vi "Write Settings.vi"(8 "error in":errorcluster, 10 "App Settings":T4, 11 "Controller in":refnum<class "Controller.lvclass">) -> (0 "error out":errorcluster, 3 "Controller out":refnum<class "Controller.lvclass">)   [LabVIEW 2022 SP3, in "Controller.lvlib" / "Controller.lvclass"]
uses:
  Controller.lvclass
  Typedefs/Storage Settings.ctl
  Typedefs/Image Formats.ctl
  Typedefs/PLC Settings.ctl
  Controller.lvclass/Controller.ctl
  <vilib>/Utility/config.llb/Write Key (U32).vi
  <vilib>/Utility/config.llb/Write Key (String).vi
  <vilib>/Utility/config.llb/Write Key (Path).vi
  <vilib>/Utility/config.llb/Write Key (Boolean).vi
  <vilib>/Utility/config.llb/NI_LVConfig.lvlib
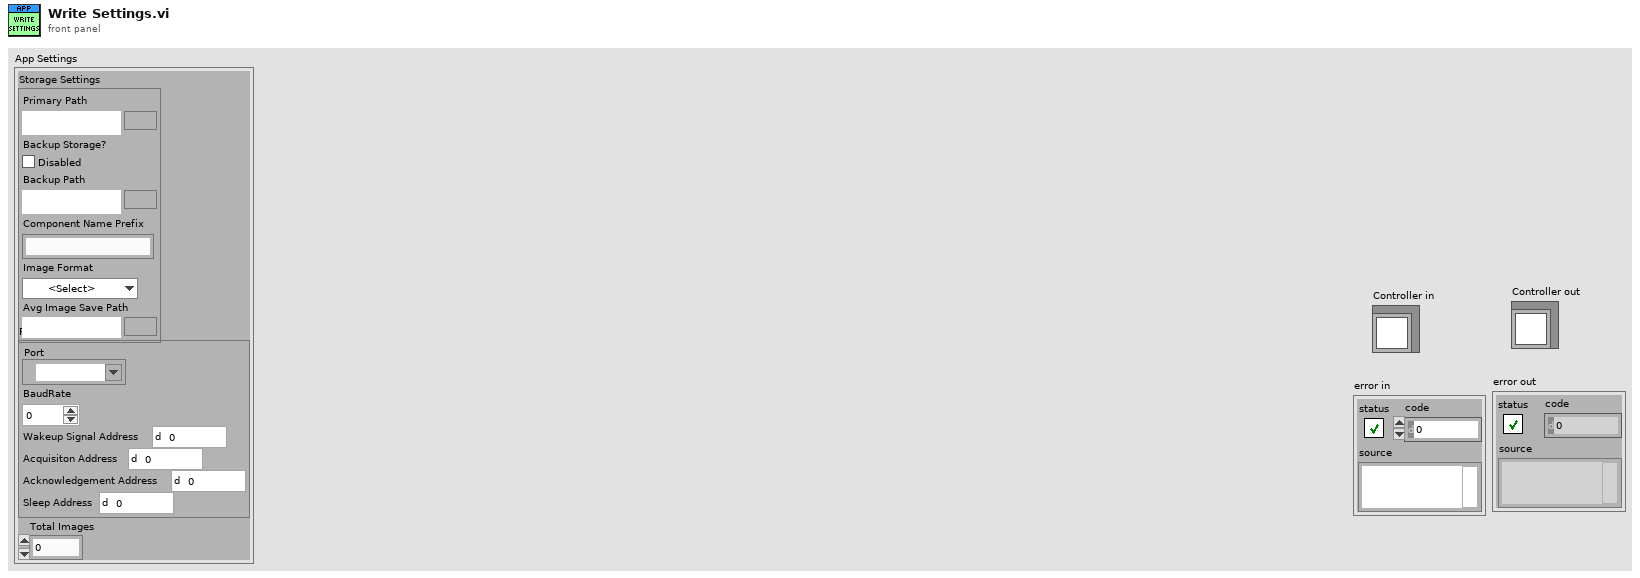
[diagram p1: front panel]
types:
  T1 = typedef "Storage Settings.ctl" = cluster{"Primary Path":path, "Backup Storage?":bool, "Backup Path":path, "Component Name Prefix":string, "Image Format":T2, "Avg Image Save Path":path}
  T2 = typedef "Image Formats.ctl" = enum16{"<Select>", "TIFF", "RAW"}
  T3 = typedef "PLC Settings.ctl" = cluster{"Port":refnum<visa-resource-name>, "BaudRate":u32, "Wakeup Signal Address ":u16, "Acquisiton Address":u16, "Acknowledgement Address":u16, "Sleep Address":u32}
  T4 = cluster{"Storage Settings":T1, "PLC Settings":T3, "Total Images":u32}
  T5 = cluster{"Config File ":path, "Configuration":path, "Event Log":path, "Error Log":path}
  T6 = typedef "NI_LVConfig.lvlib/Config Data RefNum.ctl" = refnum<k1>
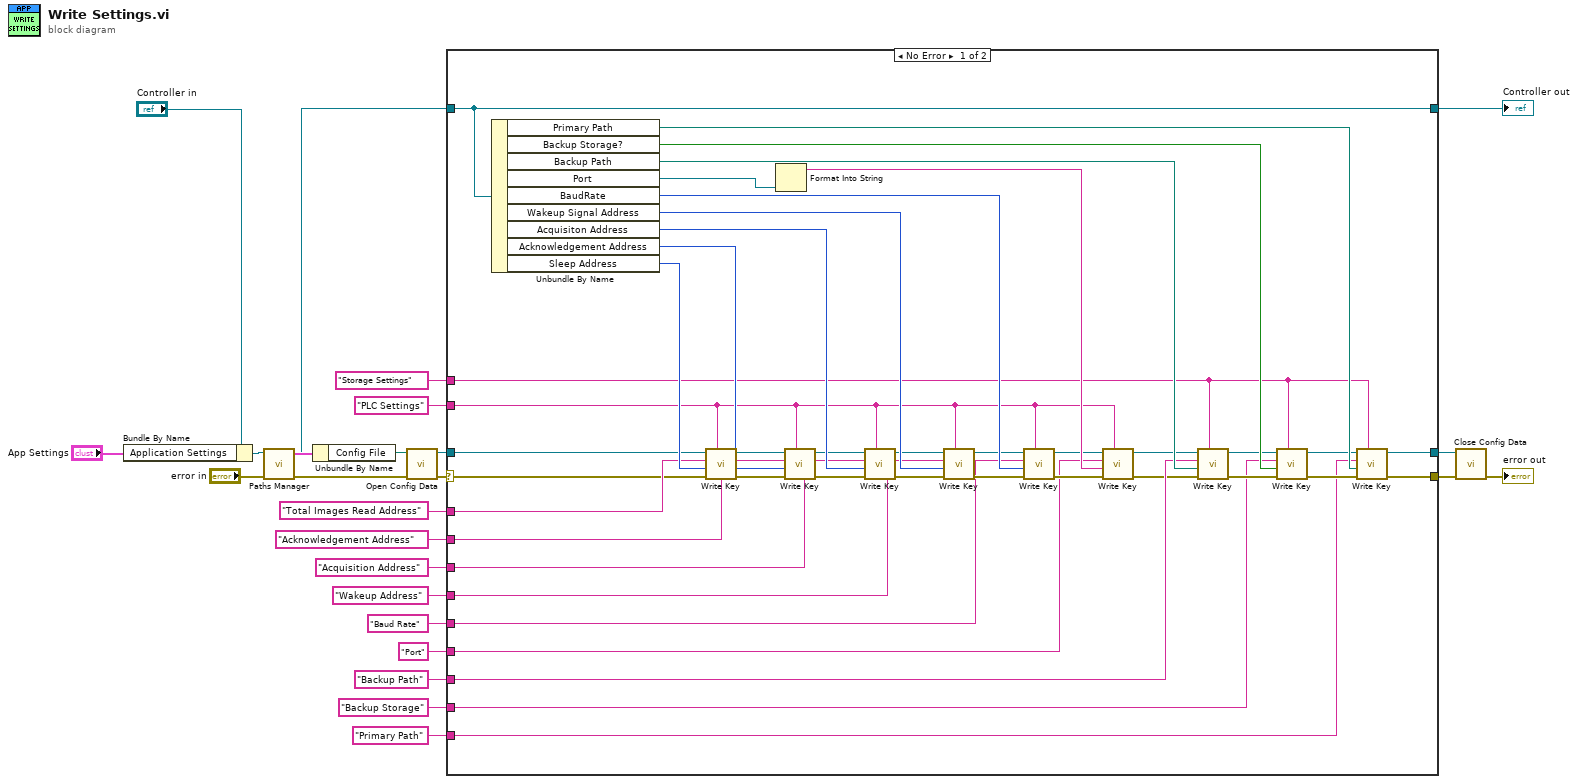
[diagram p0: block diagram]
diagram:
  n1 = Bundle By Name(cluster="Controller in", "Application Settings"="App Settings") -> (w2:refnum<class "Controller.lvclass">)
  n2 = call "Paths Manager.vi"("error in"="error in", "Controller in"=w2) -> ("error out"=w23:errorcluster, "Paths"=w21:T5, "Controller out"=w18:refnum<class "Controller.lvclass">)  [unwired: 7 in]
  n3 = Unbundle By Name(w21) -> ("Config File"=w20:path)
  n4 = call <vilib>:"Open Config Data.vi"("error in (no error)"=w23, "configuration file path"=w20) -> ("error out"=w22:errorcluster, "refnum"=w17:T6)  [unwired: 7 in, 1 out]
  n5 = case shown="No Error" w22 {
    selector: w22 -> [w29 w70]
    tunnel: [w63 w70] -> w4
    tunnel: [w30 w69] -> w25
    tunnel: w18 -> [w30 w69]
    tunnel: w17 -> [w28 w68]
    tunnel: "Storage Settings" -> [w42 _]
    tunnel: "PLC Settings" -> [w41 _]
    tunnel: "Primary Path" -> [w40 _]
    tunnel: "Backup Storage" -> [w39 _]
    tunnel: "Backup Path" -> [w38 _]
    tunnel: "Port" -> [w37 _]
    tunnel: "Baud Rate" -> [w36 _]
    tunnel: "Wakeup Address" -> [w35 _]
    tunnel: "Acquisition Address" -> [w34 _]
    tunnel: "Acknowledgement Address" -> [w33 _]
    tunnel: "Total Images Read Address" -> [w32 _]
    tunnel: [w31 w68] -> w5
    frame No Error {
      n6 = Unbundle By Name(w30) -> ("Primary Path"=w59:path, "Backup Storage?"=w58:bool, "Backup Path"=w57:path, "Port"=w56:refnum<visa-resource-name>, "BaudRate"=w54:u32, "Wakeup Signal Address"=w53:u16, "Acquisiton Address"=w52:u16, "Acknowledgement Address"=w51:u16, "Sleep Address"=w50:u32)
      n7 = call-poly <vilib>:"Write Key.vi"("section"=w41, "error in (no error)"=w29, "value"=w50, "key"=w32, "refnum"=w28) -> ("error out"=w64:errorcluster, "refnum out"=w49:T6)  [unwired: 4 in, 1 out]
      n8 = Format Into String(w56) -> (resulting string=w55:string)  [unwired: 3 in, 1 out]
      n9 = call-poly <vilib>:"Write Key.vi"("section"=w41, "error in (no error)"=w64, "value"=w51, "key"=w33, "refnum"=w49) -> ("error out"=w62:errorcluster, "refnum out"=w48:T6)  [unwired: 4 in, 1 out]
      n10 = call-poly <vilib>:"Write Key.vi"("section"=w41, "error in (no error)"=w62, "value"=w52, "key"=w34, "refnum"=w48) -> ("error out"=w67:errorcluster, "refnum out"=w47:T6)  [unwired: 4 in, 1 out]
      n11 = call-poly <vilib>:"Write Key.vi"("section"=w41, "error in (no error)"=w67, "value"=w53, "key"=w35, "refnum"=w47) -> ("error out"=w61:errorcluster, "refnum out"=w46:T6)  [unwired: 4 in, 1 out]
      n12 = call-poly <vilib>:"Write Key.vi"("section"=w41, "error in (no error)"=w61, "value"=w54, "key"=w36, "refnum"=w46) -> ("error out"=w65:errorcluster, "refnum out"=w45:T6)  [unwired: 4 in, 1 out]
      n13 = call-poly <vilib>:"Write Key.vi"("section"=w41, "error in (no error)"=w65, "value"=w55, "key"=w37, "refnum"=w45) -> ("error out"=w27:errorcluster, "refnum out"=w26:T6)  [unwired: 4 in, 1 out]
      n14 = call-poly <vilib>:"Write Key.vi"("section"=w42, "error in (no error)"=w27, "value"=w57, "key"=w38, "refnum"=w26) -> ("error out"=w60:errorcluster, "refnum out"=w44:T6)  [unwired: 4 in, 1 out]
      n15 = call-poly <vilib>:"Write Key.vi"("section"=w42, "error in (no error)"=w60, "value"=w58, "key"=w39, "refnum"=w44) -> ("error out"=w66:errorcluster, "refnum out"=w43:T6)  [unwired: 4 in, 1 out]
      n16 = call-poly <vilib>:"Write Key.vi"("section"=w42, "error in (no error)"=w66, "value"=w59, "key"=w40, "refnum"=w43) -> ("error out"=w63:errorcluster, "refnum out"=w31:T6)  [unwired: 4 in, 1 out]
    }
    frame Error {
    }
  }
  "Controller out" <- w25
  n17 = call <vilib>:"Close Config Data.vi"("error in (no error)"=w4, "refnum"=w5) -> ("error out"=→"error out":errorcluster)  [unwired: 8 in, 1 out]
